vi "Event handler-Exit.vi"(9 "Restart (F)":bool, 11 "UI queue":refnum<queue>) -> (0 "error out":errorcluster, 3 "Cancelled":bool)   [LabVIEW 2017]
uses:
  Queue/Message Queue/Typedefs/Message Cluster.ctl
  Typedefs/Frame Size.ctl
  Global Variables/gl_UI Ctrl Refs.vi
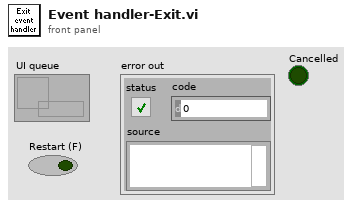
[diagram p1: front panel]
types:
  T1 = typedef "UI ctrl refs cluster.ctl" = cluster{"Top level VI path":path, "Top level VI ref":refnum<vi>, "User menu ref":refnum<k9>, "Sub Panel control":refnum<vi>, "Imaging Param Tab":refnum<vi>, "Occurrence-Start drivers":refnum<k4>, "Occurrence-Speed logging initialised":refnum<k4>, "Occurrence-XYZ stage initialised":refnum<k4>, "Exit button":refnum<vi>, "Status ind":refnum<vi>, "Set as origin":refnum<vi>, "Speed Logging":refnum<vi>, "Time Lapse":refnum<vi>, "Live Imaging":refnum<vi>, "AOL Z Stack":refnum<vi>, "Motor Z Stack":refnum<vi>, "Funct Acq button":refnum<vi>, "Hard Shutter":refnum<vi>, "Virtual Shutter":refnum<vi>, "Laser Power":refnum<vi>, "AOL Mode":refnum<vi>, "Frame Size":refnum<vi>, "Field of View":refnum<vi>, "Dwell Time":refnum<vi>, "Zoom":refnum<vi>, "AOL Z":refnum<vi>, "Objective":refnum<vi>, "Axis":refnum<vi>, "Paths & Names":refnum<vi>, "Experiment folder path (ind.)":refnum<vi>, "Last State (Ind.)":refnum<vi>, "Laser wavelength ind (nm)":refnum<vi>, "Averages":refnum<vi>, "Angle (degrees)":refnum<vi>, "X centre":refnum<vi>, "Y centre":refnum<vi>, "Plane Mode":refnum<vi>, "# Planes":refnum<vi>, "Z Start":refnum<vi>, "Z Stop":refnum<vi>, "Z Step":refnum<vi>, "PMT 1":refnum<vi>, "PMT 2":refnum<vi>, "Stage XYZ Position":refnum<vi>, "Pockels@Z Start":refnum<vi>, "Pockels@Z Stop":refnum<vi>, "Obtain Z Start":refnum<vi>, "Obtain Z Stop":refnum<vi>, "Live stim.trig.period":refnum<vi>, "Live stim.trig.enable":refnum<vi>, "Movement Correction":refnum<vi>, "Load Reference Image":refnum<vi>, "XY Stage Move":refnum<vi>, "MovCor Cluster":refnum<vi>, "RefDAQParam":refnum<vi>, "Funct. Acq. Pockels Modulation":refnum<vi>, "Background MovCor":refnum<vi>, "Ref Laser Power":refnum<vi>, "Enable Video Recording":refnum<vi>, "Video Record-Live Imaging":refnum<vi>, "Video Record-Funct acq":refnum<vi>, "Reference Source":refnum<vi>, "AOL Z-stack Chirps Ready (ind)":refnum<vi>, "Target time between mov.cor. ref triggers (ms)":refnum<vi>, "Funct. Acq. Ref frame save":refnum<vi>, "Tracking button":refnum<vi>, "Show ref plots window":refnum<vi>, "Center freq ind (nm)":refnum<vi>, "Pickup mode (ind)":refnum<vi>, "Logging queue (ind)":refnum<vi>, "Back aperture power (ind.)":refnum<vi>, "Power after objective (ind.)":refnum<vi>, "Switch user":refnum<vi>}
  T2 = typedef "Frame Size.ctl" = u16
  T3 = typedef "AOL_Globals.ctl" = cluster{"Imaging Protocol":T4, "Number of POI":u16, "Number of Miniscans":u16, "Number of Trials":u16, "Number of Cycles ":u64, "# Averaged Frames":u16, "Laser power (%)":u8, "Pockels":dbl, "Acquisition Length (sec)":dbl, "Fill time (us)":dbl, "POI Dwell time (us)":dbl, "Miniscan Dwell time per pixel (us)":dbl, "PMT 1":dbl, "PMT 2":dbl, "Back Apperture":dbl, "Frame Size":T2, "Center Frequency":dbl, "Field of View":dbl, "DwellTime (us)":dbl, "Wavelength (nm)":dbl, "Zoom":dbl, "AOL Z":dbl, "AOL Mode":T5, "GridXY":dbl, "GridZ":dbl, "TriggerPeriod (sec)":dbl, "Number of Pixels in Miniscan":u16, "Experiment folder path":path, "X centre":dbl, "Y centre":dbl, "Angle (degrees)":dbl, "Plane Mode":T6, "Threshold":u16[], "Regenerate Chirps":bool, "Rectangle ROI length (pixels)":u16, "Rectangle ROI height (pixels)":u16, "AOD fill":u16, "StartupDelay":i32, "Samples Wait after Trigger":u16, "Slip Cycle":u32, "Add Cycle":bool}
  T4 = typedef "Imaging Protocols enum.ctl" = enum16{"AOL Z-Stack", "Motor Z Stack", "Functional Acquisition", "Single Plane Acquisition", "Volume Acquisition", "Live Imaging", "Live Plane Imaging", "Live Volume Imaging"}
  T5 = typedef "AOL modes.ctl" = enum16{"Raster", "Structural", "Pointing", "Mini Scan", "Alignment"}
  T6 = typedef "Plane Mode.ctl" = u16
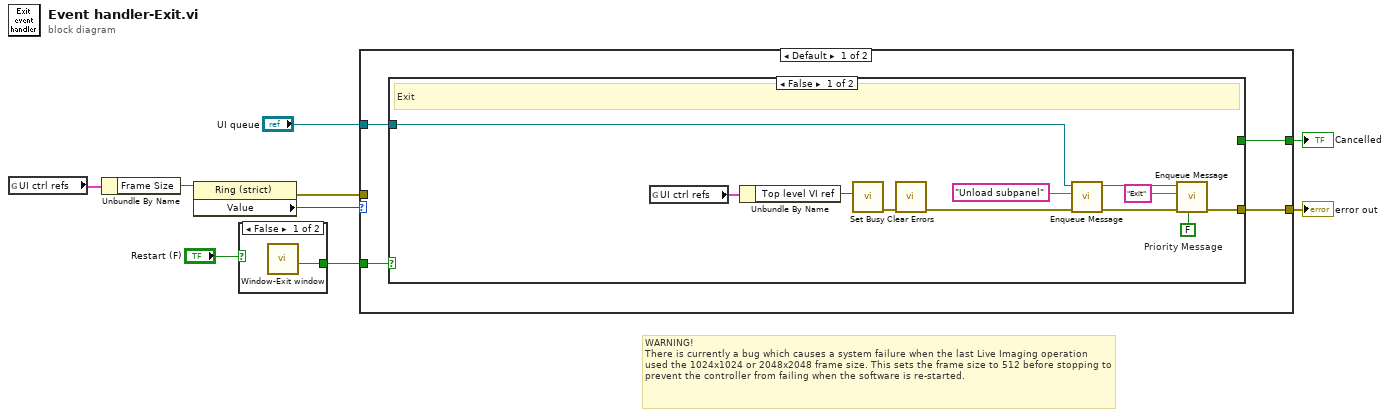
[diagram p0: block diagram]
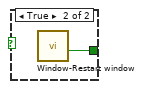
[diagram p2: hidden frame]
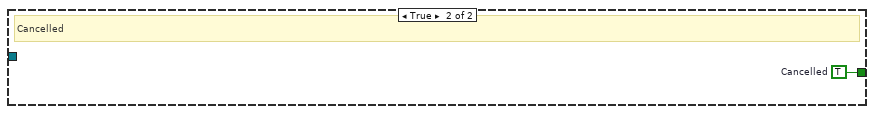
[diagram p3: hidden frame]
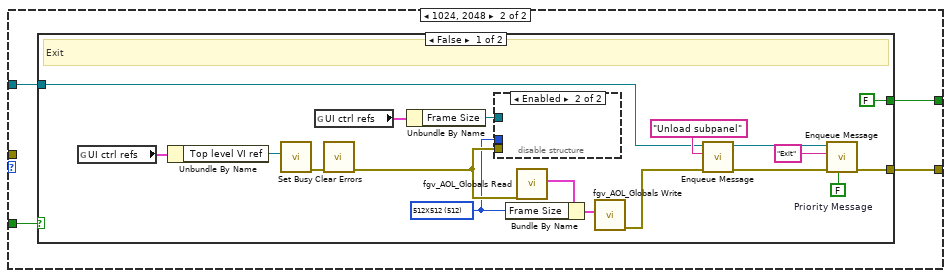
[diagram p4: hidden frame]
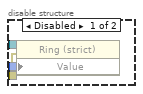
[diagram p5: hidden frame]
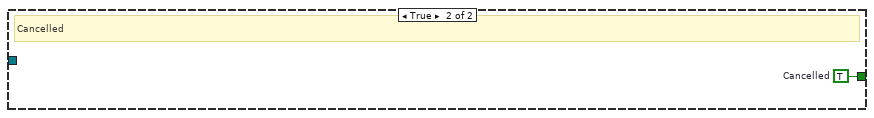
[diagram p6: hidden frame]
diagram:
  # "WARNING!\nThere is currently a bug which causes a system failure when the last Live Imaging operation used the 1024x1024 or 2048x2048 frame size. This sets the frame size to 512 before stopping to prevent the controller from failing when the software is re-started."
  n1 = global read "gl_UI Ctrl Refs.vi" "UI ctrl refs"() -> (w7:T1)
  n2 = Unbundle By Name(w7) -> ("Frame Size"=w6:refnum<vi>)
  n3 = property on="Property Node" class="Ring (strict)"(reference=w6) -> (error out=w5:errorcluster, "Value"=w4:u16)  [unwired: 1 in, 1 out]
  n4 = case shown="False" "Restart (F)" {
    tunnel: [w10 w11] -> w2
    frame False {
      n5 = call "Window-Exit window.vi"() -> ("Cancelled (Left button pressed)"=w10:bool)  [unwired: 10 in, 1 out]
    }
    frame True {
      n6 = call "Window-Restart window.vi"() -> ("Cancelled (Left button pressed)"=w11:bool)  [unwired: 10 in, 1 out]
    }
  }
  n7 = case shown="Default" w4 {
    tunnel: "UI queue" -> [w15 w31]
    tunnel: [w14 w30] -> w8
    tunnel: w5 -> [_ _]
    tunnel: [w13 w29] -> w3
    tunnel: w2 -> [w12 w28]
    frame Default {
      n8 = case shown="False" w12 {
        tunnel: [w21 _] -> w14
        tunnel: w15 -> [w17 _]
        tunnel: [_ w27] -> w13
        frame False {
          w25 = FALSE  # Priority Message
          # "Exit"
          n9 = global read "gl_UI Ctrl Refs.vi" "UI ctrl refs"() -> (w24:T1)
          n10 = Unbundle By Name(w24) -> ("Top level VI ref"=w23:refnum<vi>)
          n11 = call <vilib>:"Set Busy.vi"("VI reference (current VI)"=w23) -> ("error out"=w22:errorcluster)  [unwired: 9 in, 1 out]
          n12 = call <vilib>:"Clear Errors.vi"("error in (no error)"=w22) -> ("error out"=w18:errorcluster)  [unwired: 5 in, 1 out]
          n13 = call "Enqueue Message.vi"("error in (no error)"=w18, "Message"="Unload subpanel", "Queue"=w17) -> ("error out"=w19:errorcluster, "Queue out"=w16:refnum<queue>)  [unwired: 7 in]
          n14 = call "Enqueue Message.vi"("Priority Message? (F)"=w25, "error in (no error)"=w19, "Message"="Exit", "Queue"=w16) -> ("error out"=w21:errorcluster)  [unwired: 6 in, 1 out]
        }
        frame True {
          w27 = TRUE  # Cancelled
          # "Cancelled"
        }
      }
    }
    frame 1024, 2048 {
      n15 = case shown="False" w28 {
        tunnel: [w45 _] -> w30
        tunnel: w31 -> [w33 _]
        tunnel: [FALSE w53] -> w29
        frame False {
          w39 = T2 512 items=["100X100"=100, "128X128"=128, "200X200"=200, "256X256"=256, "512X512"=512, "1024x1024"=1024, "2048x2048"=2048] ("Value (Signaling)")
          w35 = FALSE  # Priority Message
          # "Exit"
          n16 = global read "gl_UI Ctrl Refs.vi" "UI ctrl refs"() -> (w48:T1)
          n17 = Unbundle By Name(w48) -> ("Top level VI ref"=w47:refnum<vi>)
          n18 = call <vilib>:"Set Busy.vi"("VI reference (current VI)"=w47) -> ("error out"=w46:errorcluster)  [unwired: 9 in, 1 out]
          n19 = global read "gl_UI Ctrl Refs.vi" "UI ctrl refs"() -> (w44:T1)
          n20 = call <vilib>:"Clear Errors.vi"("error in (no error)"=w46) -> ("error out"=w40:errorcluster)  [unwired: 5 in, 1 out]
          n21 = Unbundle By Name(w44) -> ("Frame Size"=w43:refnum<vi>)
          n22 = disable-structure shown="Enabled" {
            disable-tunnel: w43 -> [w52 _]
            disable-tunnel: w40 -> [w51 _]
            disable-tunnel: w39 -> [w50 _]
            frame Disabled {
              n23 = property on="Property Node" class="Ring (strict)"(reference=w52, error in=w51, "Value"=w50) -> ()  [unwired: 2 out]
            }
            frame Enabled {
            }
          }
          n24 = call "fgv_AOL_Globals Read.vi"("error in (no error)"=w40) -> ("AOL_Globals"=w42:T3)  [unwired: 8 in, 2 out]
          n25 = Bundle By Name(cluster=w42, "Frame Size"=w39) -> (w41:T3)
          n26 = call "fgv_AOL_Globals Write.vi"("AOL_Globals"=w41) -> ("error out"=w36:errorcluster)  [unwired: 10 in]
          n27 = call "Enqueue Message.vi"("error in (no error)"=w36, "Message"="Unload subpanel", "Queue"=w33) -> ("error out"=w34:errorcluster, "Queue out"=w32:refnum<queue>)  [unwired: 7 in]
          n28 = call "Enqueue Message.vi"("Priority Message? (F)"=w35, "error in (no error)"=w34, "Message"="Exit", "Queue"=w32) -> ("error out"=w45:errorcluster)  [unwired: 6 in, 1 out]
        }
        frame True {
          w53 = TRUE  # Cancelled
          # "Cancelled"
        }
      }
    }
  }
  "error out" <- w8
  "Cancelled" <- w3
